vi "3D-SaveOtherParams.vi"(8 "Param Set":cluster{"StrVel":string, "MaxVel":string}, 11 "created path":path) -> ()   [LabVIEW 2015]
uses:
  <vilib>/Utility/file.llb/Write To Spreadsheet File (string).vi
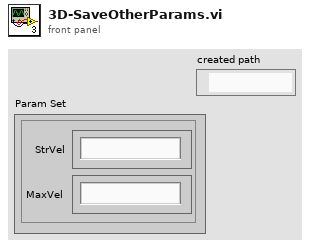
[diagram p1: front panel]
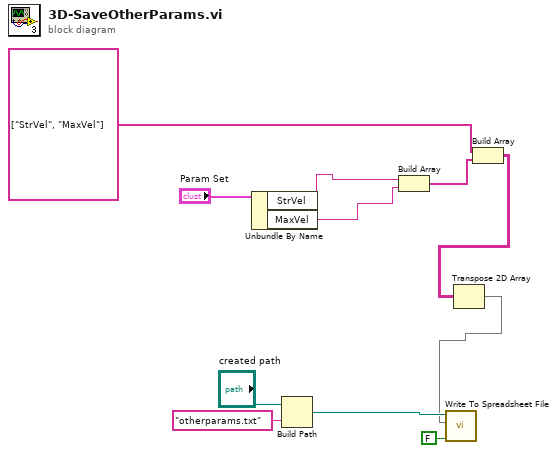
[diagram p0: block diagram]
diagram:
  n1 = Unbundle By Name("Param Set") -> ("StrVel"=w6:string, "MaxVel"=w5:string)
  n2 = Build Path(base path="created path", name or relative path="otherparams.txt" ("名称或相对路径")) -> (appended path=w9:path)
  n3 = Build Array(w6, w5) -> (w3:string[])
  n4 = Build Array(string[] ["StrVel", "MaxVel"], w3) -> (w2:string[][])
  n5 = Transpose 2D Array(2D array=w2) -> (transposed array=w1:string[][])
  n6 = call-poly <vilib>:"Write To Spreadsheet File.vi"("append to file? (new file:F)"=FALSE, "2D data"=w1, "file path (dialog if empty)"=w9) -> ()  [unwired: 5 in, 1 out]
